vi "Get Pot Zero.vi"() -> (2 "Left Pot 0":dbl, 3 "Right Pot 0":dbl)   [LabVIEW 2014]
uses:
  Robot Global Data.vi
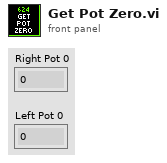
[diagram p1: front panel]
types:
  T1 = typedef "Dashboard Control Data.ctl" = cluster{"Cam Exposure":dbl, "Go to angle":dbl, "Steer PID Gains":cluster{"proportional gain (Kc)":dbl, "integral time (Ti, min)":dbl, "derivative time (Td, min)":dbl}, "Steer PID output Range":cluster{"output high":dbl, "output low":dbl}, "Pressure m \nValue":dbl, "Pressure b \nValue":dbl, "Strafe Timer\nWait":dbl, "Roller Command Cluster ":T2, "Elevator":T3, "Strafe Correct min X":dbl, "IMU Enable":bool, "Encoder Control":T5}
  T2 = typedef "Roller Control.ctl" = cluster{"Left Roller Speed":dbl, "Right Roller Speed":dbl, "Left Roller Speed Back":dbl, "Right Roller Speed Back":dbl, "Roller Align Decide Limit":u32, "Left Roller Speed Unload":dbl, "Right Roller Speed Unload":dbl, "Ping Dist Difference":dbl, "Ping In Dist":dbl, "Right Pot 0":dbl, "Pot Threshold":dbl, "Left Pot 0":dbl, "Manual 0s?":bool, "Right Pot Scale":dbl, "Left Pot Scale":dbl, "0 wait time":i32, "Reset?":bool}
  T3 = typedef "Elevator DB Control.ctl" = cluster{"PID Output Range":cluster{"output high":dbl, "output low":dbl}, "PID gains":cluster{"proportional gain (Kc)":dbl, "integral time (Ti, min)":dbl, "derivative time (Td, min)":dbl}, "Height Tolerance":dbl, " Encoder Constant":dbl, "Safe Mode Max Speed":dbl, "Eject Time":dbl, "Encoder Filter?":bool, "Zeroing Speed":dbl, "Presets":T4}
  T4 = typedef "Elevator Presets.ctl" = cluster{"Hold Tote":dbl, "Hold Trashcan":dbl, "Pickup 2 w/ Tote":dbl, "Pickup 2 w/ Trashcan":dbl, "Pickup 3 w/ Tote":dbl, "Pickup 3 w/ Trashcan":dbl, "Bottom":dbl, "Pickup 1 w/ Tote":dbl, "Pickup Trashcan":dbl, "Pickup 1 w/ Trashcan":dbl, "Eject":dbl}
  T5 = typedef "Encoder Control.ctl" = cluster{"Left Tick Constant":dbl, "Right Tick Constant":dbl, "Center Tick Constant":dbl, "Reset?":bool}
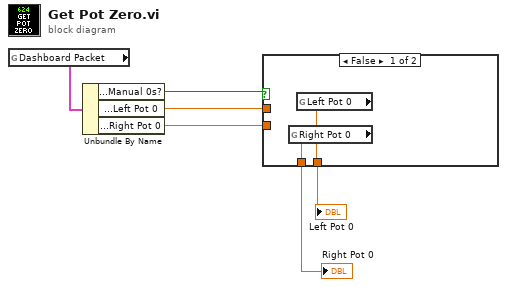
[diagram p0: block diagram]
diagram:
  n1 = global read "Robot Global Data.vi" "Dashboard Packet"() -> (w4:T1)
  n2 = Unbundle By Name(w4) -> ("Roller Command Cluster.Manual 0s?"=w3:bool, "Roller Command Cluster.Left Pot 0"=w2:dbl, "Roller Command Cluster.Right Pot 0"=w1:dbl)
  n3 = case shown="False" w3 {
    tunnel: [w7 w10] -> w5
    tunnel: [w8 w9] -> w6
    tunnel: w2 -> [_ w10]
    tunnel: w1 -> [_ w9]
    frame False {
      n4 = global read "Robot Global Data.vi" "Right Pot 0"() -> (w8:dbl)
      n5 = global read "Robot Global Data.vi" "Left Pot 0"() -> (w7:dbl)
    }
    frame True {
    }
  }
  "Right Pot 0" <- w6
  "Left Pot 0" <- w5
